vi "Ch1-Ex5.vi"() -> ()   [LabVIEW 2018]
panel:
  out "Triggered":bool
  in  "Numeric":dbl
  in  "Slide":dbl(slide) scale=0.0..10.0
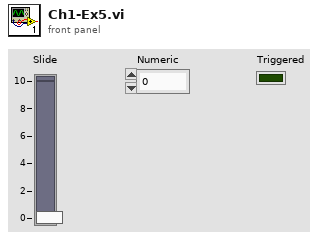
[diagram p1: front panel]
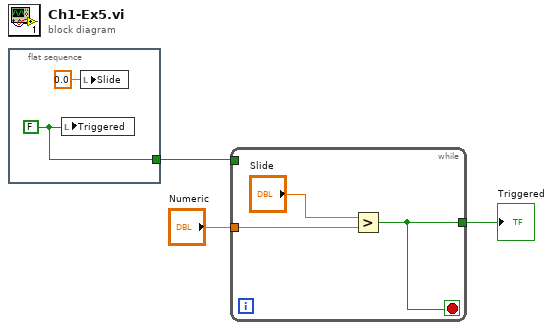
[diagram p0: block diagram]
diagram:
  n1 = flat-sequence {
    tunnel: [w4] -> w1
    frame #0 {
      w4 = FALSE ("Triggered")
      n2 = local write "Triggered"(w4) -> ()
      n3 = local write "Slide"(0.0 ("Slide")) -> ()
    }
  }
  n4 = while {
    tunnel: "Numeric" -> [w7]
    tunnel: [w6] -> w2
    tunnel: w1 -> [_]
    stop <- w6 stop-if-true
    n5 = Greater?(x="Slide", y=w7) -> (0:w6:bool)
  }
  "Triggered" <- w2
